vi "Create NetworkStream Connection.vi"(5 "Connection.NetworkStream":refnum<class "Connection.NetworkStream.lvclass">, 8 "error in (no error)":errorcluster, 9 "Stream Name":string, 10 "Outbound":refnum<k21>, 11 "Inbound":refnum<k21>) -> (0 "error out":errorcluster, 3 "Connection.NetworkStream":refnum<class "Connection.NetworkStream.lvclass">)   [LabVIEW 2013, in "Connection.NetworkQueue_GOSPL.lvlib" / "Connection.NetworkStream.lvclass"]
uses:
  Connection.NetworkStream/Connection.NetworkStream.lvclass
  Connection.NetworkStream/Connection.NetworkStream.lvclass/Connection.NetworkStream.ctl
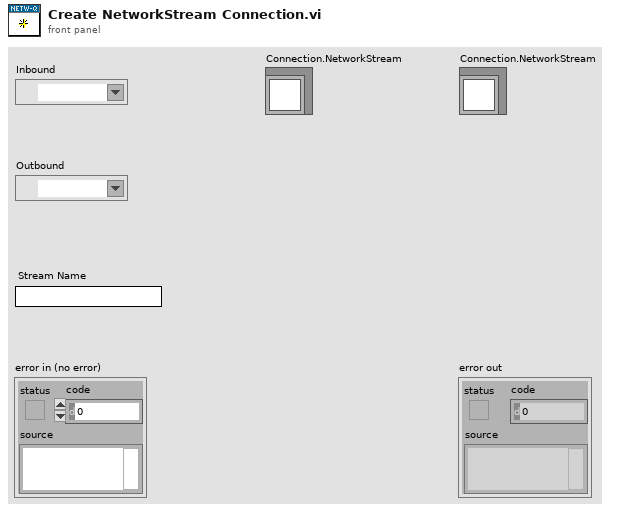
[diagram p1: front panel]
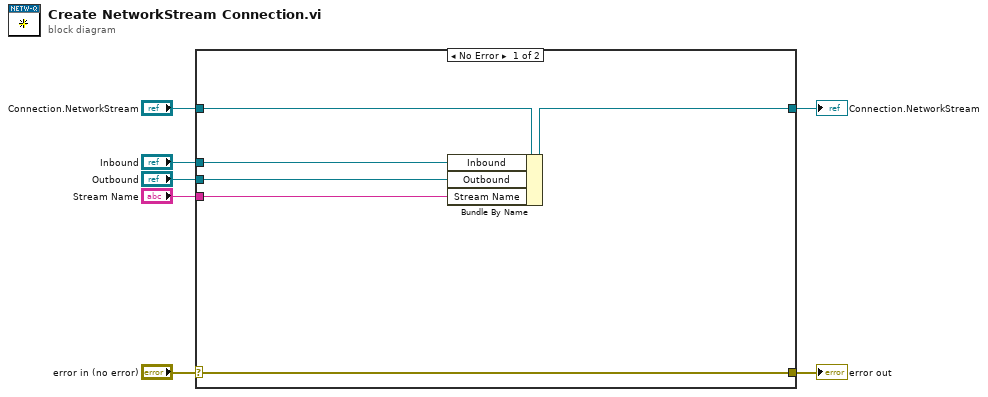
[diagram p0: block diagram]
diagram:
  n1 = case shown="No Error" "error in (no error)" {
    selector: "error in (no error)" -> [w12 w15]
    tunnel: [w12 w15] -> w6
    tunnel: [w11 w14] -> w4
    tunnel: "Connection.NetworkStream" -> [w13 w14]
    tunnel: "Inbound" -> [w10 _]
    tunnel: "Stream Name" -> [w9 _]
    tunnel: "Outbound" -> [w8 _]
    frame No Error {
      n2 = Bundle By Name(cluster=w13, "Inbound"=w10, "Outbound"=w8, "Stream Name"=w9) -> (w11:refnum<class "Connection.NetworkStream.lvclass">)
    }
    frame Error {
    }
  }
  "error out" <- w6
  "Connection.NetworkStream" <- w4
